vi "Test Coffee Shop Barista Registers With Order Queue When Added.vi"(8 "error in (no error)":errorcluster, 11 "Coffee Shop Test in":refnum<class "Coffee Shop Test.lvclass">=refnum) -> (0 "error out":errorcluster, 3 "Coffee Shop Test out":refnum<class "Coffee Shop Test.lvclass">)   [LabVIEW 2020, in "Coffee Shop Test.lvclass"]
uses:
  Coffee Shop Test.lvclass
  <vilib>/Astemes/Triarc Framework/Process/Process.lvclass
  Processes/Coffee Shop/Coffee Shop.lvclass
  Test Doubles/Mock Job Handler/Mock Job Handler.lvclass
  C:/Program Files (x86)/National Instruments/LabVIEW 2020/vi.lib/Astemes/Triarc Framework/Application/Application.lvclass
  C:/Program Files (x86)/National Instruments/LabVIEW 2020/vi.lib/Astemes/Triarc Framework/Process/Process.lvclass
  C:/Program Files (x86)/National Instruments/LabVIEW 2020/vi.lib/Astemes/Triarc Framework/Base/Base.lvclass
  C:/Program Files (x86)/National Instruments/LabVIEW 2020/vi.lib/Astemes/Triarc Framework/Error Handler Interface/Error Handler Interface.lvclass
  C:/Program Files (x86)/National Instruments/LabVIEW 2020/vi.lib/Astemes/Triarc Framework/Logging/Logging.lvclass
  C:/Program Files (x86)/National Instruments/LabVIEW 2020/vi.lib/Astemes/Triarc Framework/Async Handler/Async Handler.lvclass
  C:/git/astemes-triarc-examples/source/Coffee Shop/Processes/Coffee Shop/Coffee Shop.lvclass
  Processes/People/Person/Person.lvclass
  87fb295b-fc3e-4637-b8c5-7bb4b2509809.vi
  <vilib>/Astemes/LUnit/Test Case.lvclass
  C:/Program Files (x86)/National Instruments/LabVIEW 2020/vi.lib/Astemes/LUnit/Test Case.lvclass
  C:/Program Files (x86)/National Instruments/LabVIEW 2020/vi.lib/Astemes/LUnit/LUnit Runnable.lvclass
  C:/git/astemes-triarc-examples/source/Coffee Shop/Tests/Test Doubles/Mock Job Handler/Mock Job Handler.lvclass
  C:/git/astemes-triarc-examples/source/Coffee Shop/Processes/People/Process Job/Job Handler.lvclass
  C:/Program Files (x86)/National Instruments/LabVIEW 2020/vi.lib/Astemes/Triarc Framework/View/View.lvclass
  C:/git/astemes-triarc-examples/source/Coffee Shop/Processes/People/Person/Person.lvclass
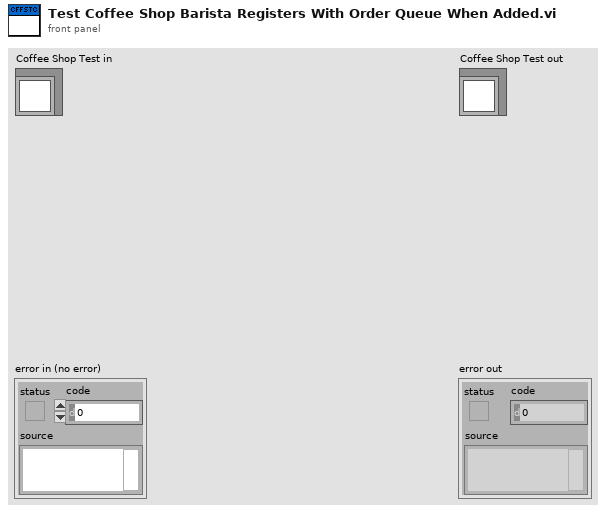
[diagram p1: front panel]
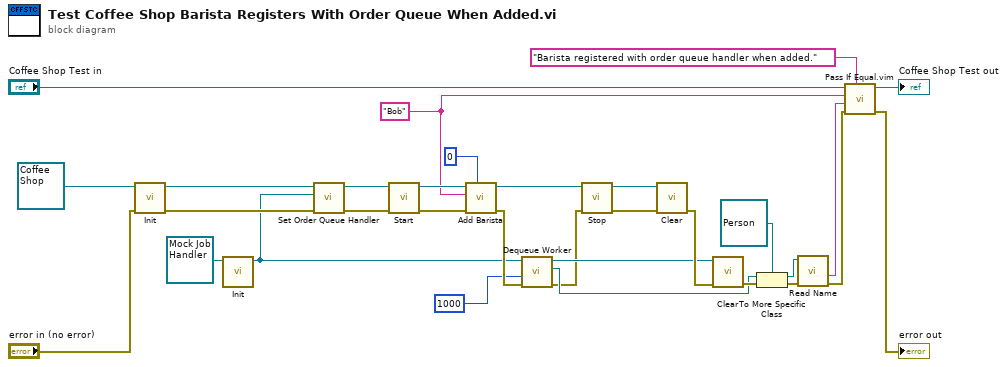
[diagram p0: block diagram]
diagram:
  w4 = "Bob" ("Name")
  n1 = call-dynamic "Init.vi"("error in (no error)"="error in (no error)", "Process In"=refnum<class "Coffee Shop.lvclass"> refnum ("Coffee Shop.lvclass")) -> ("error out"=w30:errorcluster, "Process Out"=w23:refnum<class "Coffee Shop.lvclass">)  [unwired: 8 in]
  n2 = call-dynamic "Init.vi"("Mock Job Handler In"=refnum<class "Mock Job Handler.lvclass"> refnum) -> ("Mock Job Handler Out"=w1:refnum<class "Mock Job Handler.lvclass">)  [unwired: 9 in, 1 out]
  n3 = call "Set Order Queue Handler.vi"("error in (no error)"=w30, "Order Queue Handler"=w1, "Coffee Shop In"=w23) -> ("error out"=w28:errorcluster, "Coffee Shop Out"=w29:refnum<class "Coffee Shop.lvclass">)  [unwired: 7 in]
  n4 = call <vilib>:"Start.vi"("error in (no error)"=w28, "Process In"=w29) -> ("error out"=w27:errorcluster, "Process Out"=w22:refnum<class "Coffee Shop.lvclass">)  [unwired: 7 in, 1 out]
  n5 = call "Add Barista.vi"("Time Scale [ms]"=u32 0, "error in (no error)"=w27, "Name"=w4, "Coffee Shop in"=w22) -> ("error out"=w19:errorcluster, "Coffee Shop out"=w21:refnum<class "Coffee Shop.lvclass">)  [unwired: 6 in]
  n6 = call "Dequeue Worker.vi"("error in (no error)"=w19, "timeout in ms (-1)"=1000, "Mock Job Handler In"=w1) -> ("error out"=w8:errorcluster, "element"=w10:refnum<class "Job Handler.lvclass">, "Mock Job Handler Out"=w17:refnum<class "Mock Job Handler.lvclass">)  [unwired: 5 in, 1 out]
  n7 = call <vilib>:"Stop.vi"("error in (no error)"=w8, "Process In"=w21) -> ("error out"=w25:errorcluster, "Process Out"=w26:refnum<class "Coffee Shop.lvclass">)  [unwired: 7 in, 1 out]
  n8 = call-dynamic "Clear.vi"("error in (no error)"=w25, "Application In"=w26) -> ("error out"=w18:errorcluster)  [unwired: 9 in]
  n9 = call-dynamic "Clear.vi"("error in (no error)"=w18, "Mock Job Handler In"=w17) -> ("error out"=w12:errorcluster)  [unwired: 9 in]
  n10 = To More Specific Class(target class=refnum<class "Person.lvclass"> refnum ("Process In"), reference=w10) -> (specific class reference=w6:refnum<class "Person.lvclass">)  [unwired: 1 in, 1 out]
  n11 = call <vilib>:"Read Name.vi"("error in (no error)"=w12, "Process In"=w6) -> ("error out"=w7:errorcluster, "Name"=w5:string)  [unwired: 6 in, 2 out]
  n12 = call "Pass If Equal.vim"("Description"="Barista registered with order queue handler when added.", "error in (no error)"=w7, "Actual"=w5, "Expected"=w4, "LUnit Test Case In"="Coffee Shop Test in") -> ("error out"=→"error out":errorcluster, "LUnit Test Case Out"=→"Coffee Shop Test out":refnum<class "Test Case.lvclass">)  [unwired: 5 in]
